vi "Plot menu activation location v2.vi"(8 "error in (no error)":errorcluster, 10 "Coords":T4, 11 "Refs":T3) -> (0 "error out":errorcluster, 2 "Location.Scale":T1, 3 "Location":T2)   [LabVIEW 2021, in "RocketPlot.lvlib"]
uses:
  RocketPlot.lvlib
  <vilib>/Utility/miscctls.llb/LVPoint32TypeDef.ctl
  TypeDefs/Plot UI references.ctl
  Classes/RocketPlotHandle/RocketPlotHandle.lvclass
  <userlib>/bjustice/TipStripOOPanel/Classes/TipPanelHandle/TipPanelHandle.lvclass
  TypeDefs/Plot top row.ctl
  Plot menu activation submenu type v2.ctl
  TypeDefs/Plot axis.ctl
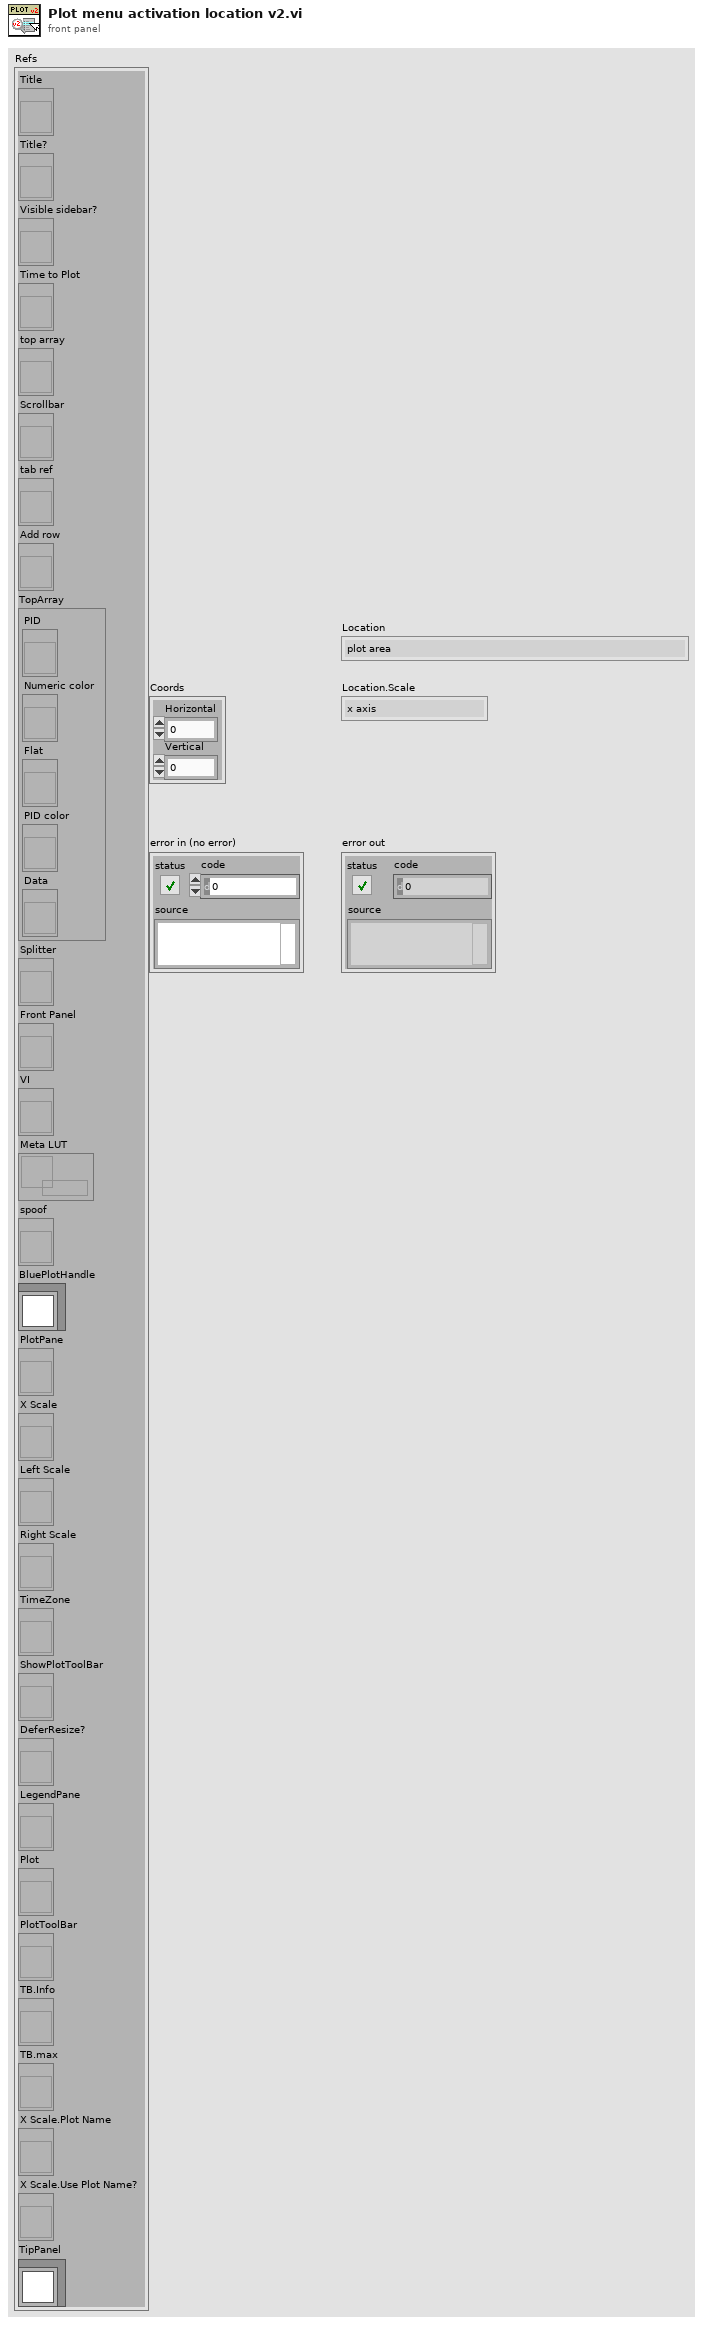
[diagram p1: front panel]
types:
  T1 = typedef "RocketPlot.lvlib/Plot axis.ctl" = enum16{"x axis", "left axis", "right axis"}
  T2 = typedef "RocketPlot.lvlib/Plot menu activation submenu type v2.ctl" = enum16{"plot area", "plot border", "markers", "scale"}
  T3 = typedef "RocketPlot.lvlib/Plot UI references.ctl" = cluster{"Title":refnum<vi>, "Title?":refnum<vi>, "Visible sidebar?":refnum<vi>, "Time to Plot":refnum<vi>, "top array":refnum<vi>, "Scrollbar":refnum<vi>, "tab ref":refnum<vi>, "Add row":refnum<vi>, "TopArray":cluster{"PID":refnum<vi>, "Numeric color":refnum<vi>, "Flat":refnum<vi>, "PID color":refnum<vi>, "Data":refnum<vi>}, "Splitter":refnum<vi>, "Front Panel":refnum<vi>, "VI":refnum<vi>, "Meta LUT":refnum<data-value>, "spoof":refnum<vi>, "BluePlotHandle":refnum<class "RocketPlotHandle.lvclass">, "PlotPane":refnum<vi>, "X Scale":refnum<vi>, "Left Scale":refnum<vi>, "Right Scale":refnum<vi>, "TimeZone":refnum<vi>, "ShowPlotToolBar":refnum<vi>, "DeferResize?":refnum<vi>, "LegendPane":refnum<vi>, "Plot":refnum<vi>, "PlotToolBar":refnum<vi>, "TB.Info":refnum<vi>, "TB.max":refnum<vi>, "X Scale.Plot Name":refnum<vi>, "X Scale.Use Plot Name?":refnum<vi>, "TipPanel":refnum<class "TipPanelHandle.lvclass">}
  T4 = typedef "LVPoint32TypeDef.ctl" = cluster{"Horizontal":i32, "Vertical":i32}
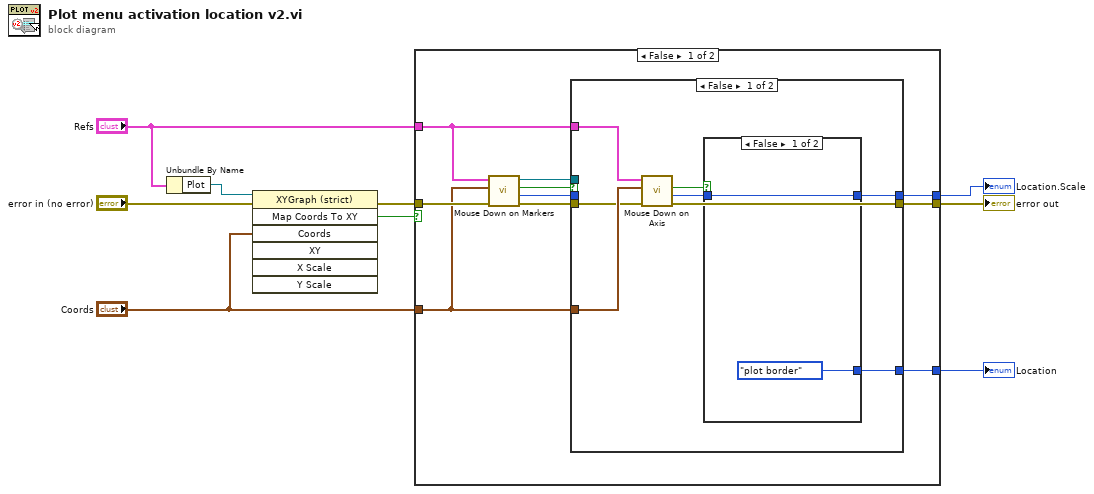
[diagram p0: block diagram]
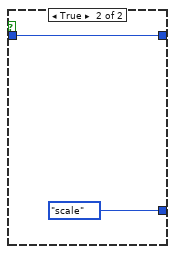
[diagram p2: hidden frame]
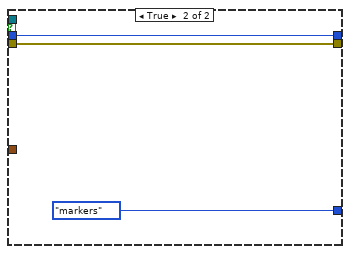
[diagram p3: hidden frame]
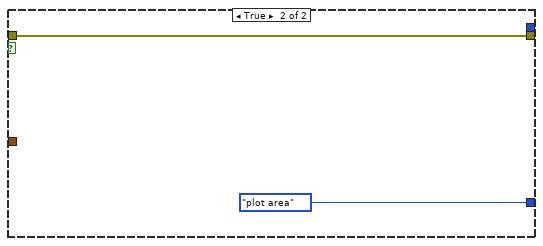
[diagram p4: hidden frame]
diagram:
  n1 = Unbundle By Name("Refs") -> ("Plot"=w3:refnum<vi>)
  n2 = invoke class="XYGraph (strict)" method="Map Coords To XY"(reference=w3, error in="error in (no error)", "Coords"="Coords") -> (error out=w4:errorcluster, "Map Coords To XY"=w1:bool)  [unwired: 4 in, 5 out]
  n3 = case shown="False" w1 {
    tunnel: [w15 Plot_menu_activation_submenu_type_v2."plot area" ("Enum")] -> w9
    tunnel: [w14 _] -> w8
    tunnel: [w13 w36] -> w7
    tunnel: "Refs" -> [w12 _]
    tunnel: w4 -> [w11 w36]
    tunnel: "Coords" -> [w10 _]
    frame False {
      n4 = call "Mouse Down on Markers.vi"("error in (no error)"=w11, "Coords"=w10, "Refs"=w12) -> ("error out"=w16:errorcluster, "target axis"=w18:T1, "Mouse down on axis marker?"=w19:bool, "ScaleRef"=w17:refnum<vi>)  [unwired: 5 in]
      n5 = case shown="False" w19 {
        tunnel: w18 -> [_ w34]
        tunnel: w10 -> [w27 _]
        tunnel: [w21 w34] -> w14
        tunnel: w12 -> [w26 _]
        tunnel: w17 -> [_ _]
        tunnel: w16 -> [w25 w32]
        tunnel: [w22 Plot_menu_activation_submenu_type_v2."markers" ("Enum")] -> w15
        tunnel: [w20 w32] -> w13
        frame False {
          n6 = call "Mouse Down on Axis.vi"("error in (no error)"=w25, "Coords"=w27, "Refs"=w26) -> ("error out"=w20:errorcluster, "target axis"=w23:T1, "Mouse down on Axis?"=w24:bool)  [unwired: 5 in, 1 out]
          n7 = case shown="False" w24 {
            tunnel: w23 -> [w29 w30]
            tunnel: [Plot_menu_activation_submenu_type_v2."plot border" ("Enum") Plot_menu_activation_submenu_type_v2."scale" ("Enum")] -> w22
            tunnel: [w29 w30] -> w21
            frame False {
            }
            frame True {
            }
          }
        }
        frame True {
        }
      }
    }
    frame True {
    }
  }
  "error out" <- w7
  "Location" <- w9
  "Location.Scale" <- w8
